vi "Controller List.vi"(11 "Controller List":T1[](array[typedef])=[{"Controller Name"=enum."Kuhnke", "CommSeg"=1, "PWM?"=TRUE, "Frequency"=100, "Low Command"=10.0, "High Command"=100.0, "Stop Command"=10.0, "Command Step"=0.1, "Solenoid Stop?"=FALSE, "Controller?"=TRUE, "Invert PWM"=TRUE, "Flange Mount Ctrl"=FALSE, "Diagnostic Mode"=enum."None"}, {"Controller Name"=enum."Helbako BLDC", "CommSeg"=1, "PWM?"=TRUE, "Frequency"=100, "Low Command"=10.0, "High Command"=100.0, "Stop Command"=10.0, "Command Step"=0.1, "Solenoid Stop?"=FALSE, "Controller?"=TRUE, "Invert PWM"=TRUE, "Flange Mount Ctrl"=FALSE, "Diagnostic Mode"=enum."None"}, {"Controller Name"=enum."Conti", "CommSeg"=1, "PWM?"=FALSE, "Frequency"=100, "Low Command"=0.0, "High Command"=800.0, "Stop Command"=0.0, "Command Step"=1.0, "Solenoid Stop?"=FALSE, "Controller?"=TRUE, "Invert PWM"=FALSE, "Flange Mount Ctrl"=FALSE, "Diagnostic Mode"=enum."None"}, {"Controller Name"=enum."Hella BLDC OL PWM", "CommSeg"=1, "PWM?"=FALSE, "Frequency"=100, "Low Command"=0.0, "High Command"=100.0, "Stop Command"=0.0, "Command Step"=0.1, "Solenoid Stop?"=FALSE, "Controller?"=TRUE, "Invert PWM"=FALSE, "Flange Mount Ctrl"=FALSE, "Diagnostic Mode"=enum."None"}, {"Controller Name"=enum."Hella BLDC Turbine OL PWM", "CommSeg"=1, "PWM?"=FALSE, "Frequency"=100, "Low Command"=0.0, "High Command"=100.0, "Stop Command"=0.0, "Command Step"=0.1, "Solenoid Stop?"=FALSE, "Controller?"=TRUE, "Invert PWM"=FALSE, "Flange Mount Ctrl"=FALSE, "Diagnostic Mode"=enum."None"}, {"Controller Name"=enum."Hella BLDC Pressure", "CommSeg"=1, "PWM?"=FALSE, "Frequency"=100, "Low Command"=0.0, "High Command"=100.0, "Stop Command"=0.0, "Command Step"=0.1, "Solenoid Stop?"=FALSE, "Controller?"=TRUE, "Invert PWM"=FALSE, "Flange Mount Ctrl"=FALSE, "Diagnostic Mode"=enum."None"}, {"Controller Name"=enum."Helbako (old)", "CommSeg"=1, "PWM?"=FALSE, "Frequency"=100, "Low Command"=0.0, "High Command"=100.0, "Stop Command"=0.0, "Command Step"=0.1, "Solenoid Stop?"=FALSE, "Controller?"=TRUE, "Invert PWM"=FALSE, "Flange Mount Ctrl"=FALSE, "Diagnostic Mode"=enum."None"}, {"Controller Name"=enum."TI PWM", "CommSeg"=1, "PWM?"=TRUE, "Frequency"=100, "Low Command"=0.0, "High Command"=100.0, "Stop Command"=0.0, "Command Step"=0.1, "Solenoid Stop?"=FALSE, "Controller?"=TRUE, "Invert PWM"=FALSE, "Flange Mount Ctrl"=FALSE, "Diagnostic Mode"=enum."None"}, {"Controller Name"=enum."PSA", "CommSeg"=1, "PWM?"=TRUE, "Frequency"=100, "Low Command"=5.0, "High Command"=95.0, "Stop Command"=5.0, "Command Step"=0.1, "Solenoid Stop?"=FALSE, "Controller?"=TRUE, "Invert PWM"=TRUE, "Flange Mount Ctrl"=TRUE, "Diagnostic Mode"=enum."PSA"}, {"Controller Name"=enum."Hella Gas", "CommSeg"=1, "PWM?"=FALSE, "Frequency"=100, "Low Command"=0.0, "High Command"=800.0, "Stop Command"=0.0, "Command Step"=1.0, "Solenoid Stop?"=TRUE, "Controller?"=TRUE, "Invert PWM"=FALSE, "Flange Mount Ctrl"=FALSE, "Diagnostic Mode"=enum."None"}, {"Controller Name"=enum."Hella Diesel", "CommSeg"=1, "PWM?"=FALSE, "Frequency"=100, "Low Command"=370.0, "High Command"=461.0, "Stop Command"=370.0, "Command Step"=1.0, "Solenoid Stop?"=TRUE, "Controller?"=TRUE, "Invert PWM"=FALSE, "Flange Mount Ctrl"=FALSE, "Diagnostic Mode"=enum."None"}, {"Controller Name"=enum."8 Comm", "CommSeg"=4, "PWM?"=FALSE, "Frequency"=100, "Low Command"=0.0, "High Command"=1.0, "Stop Command"=0.0, "Command Step"=1.0, "Solenoid Stop?"=FALSE, "Controller?"=FALSE, "Invert PWM"=FALSE, "Flange Mount Ctrl"=FALSE, "Diagnostic Mode"=enum."None"}, {"Controller Name"=enum."10 Comm", "CommSeg"=5, "PWM?"=FALSE, "Frequency"=100, "Low Command"=0.0, "High Command"=1.0, "Stop Command"=0.0, "Command Step"=1.0, "Solenoid Stop?"=FALSE, "Controller?"=FALSE, "Invert PWM"=FALSE, "Flange Mount Ctrl"=FALSE, "Diagnostic Mode"=enum."None"}, {"Controller Name"=enum."8 Comm Hella", "CommSeg"=4, "PWM?"=TRUE, "Frequency"=150, "Low Command"=0.0, "High Command"=50.0, "Stop Command"=80.0, "Command Step"=0.1, "Solenoid Stop?"=FALSE, "Controller?"=TRUE, "Invert PWM"=FALSE, "Flange Mount Ctrl"=FALSE, "Diagnostic Mode"=enum."None"}, {"Controller Name"=enum."10 Comm Hella", "CommSeg"=5, "PWM?"=TRUE, "Frequency"=150, "Low Command"=0.0, "High Command"=50.0, "Stop Command"=80.0, "Command Step"=0.1, "Solenoid Stop?"=FALSE, "Controller?"=TRUE, "Invert PWM"=FALSE, "Flange Mount Ctrl"=FALSE, "Diagnostic Mode"=enum."None"}, {"Controller Name"=enum."8 Comm Omron", "CommSeg"=4, "PWM?"=TRUE, "Frequency"=150, "Low Command"=5.0, "High Command"=50.0, "Stop Command"=75.0, "Command Step"=0.1, "Solenoid Stop?"=FALSE, "Controller?"=TRUE, "Invert PWM"=FALSE, "Flange Mount Ctrl"=FALSE, "Diagnostic Mode"=enum."None"}, {"Controller Name"=enum."10 Comm Omron", "CommSeg"=5, "PWM?"=TRUE, "Frequency"=150, "Low Command"=5.0, "High Command"=50.0, "Stop Command"=75.0, "Command Step"=0.1, "Solenoid Stop?"=FALSE, "Controller?"=TRUE, "Invert PWM"=FALSE, "Flange Mount Ctrl"=FALSE, "Diagnostic Mode"=enum."None"}, {"Controller Name"=enum."8 Comm Nissan", "CommSeg"=4, "PWM?"=TRUE, "Frequency"=10, "Low Command"=50.0, "High Command"=90.0, "Stop Command"=50.0, "Command Step"=0.1, "Solenoid Stop?"=TRUE, "Controller?"=TRUE, "Invert PWM"=FALSE, "Flange Mount Ctrl"=FALSE, "Diagnostic Mode"=enum."None"}, {"Controller Name"=enum."10 Comm Nissan", "CommSeg"=5, "PWM?"=TRUE, "Frequency"=10, "Low Command"=50.0, "High Command"=90.0, "Stop Command"=50.0, "Command Step"=0.1, "Solenoid Stop?"=TRUE, "Controller?"=TRUE, "Invert PWM"=FALSE, "Flange Mount Ctrl"=FALSE, "Diagnostic Mode"=enum."None"}, {"Controller Name"=enum."8 Comm Hella (for FCA)", "CommSeg"=4, "PWM?"=TRUE, "Frequency"=150, "Low Command"=11.0, "High Command"=89.0, "Stop Command"=10.0, "Command Step"=0.1, "Solenoid Stop?"=FALSE, "Controller?"=TRUE, "Invert PWM"=TRUE, "Flange Mount Ctrl"=FALSE, "Diagnostic Mode"=enum."None"}, {"Controller Name"=enum."Mazda BLDC", "CommSeg"=1, "PWM?"=TRUE, "Frequency"=250, "Low Command"=10.0, "High Command"=90.0, "Stop Command"=5.0, "Command Step"=0.1, "Solenoid Stop?"=FALSE, "Controller?"=TRUE, "Invert PWM"=TRUE, "Flange Mount Ctrl"=FALSE, "Diagnostic Mode"=enum."None"}, {"Controller Name"=enum."CMFB", "CommSeg"=1, "PWM?"=TRUE, "Frequency"=250, "Low Command"=0.0, "High Command"=100.0, "Stop Command"=10.0, "Command Step"=0.1, "Solenoid Stop?"=FALSE, "Controller?"=TRUE, "Invert PWM"=TRUE, "Flange Mount Ctrl"=TRUE, "Diagnostic Mode"=enum."CMFB"}]) -> (3 "Controller List OUT":T1[](array[typedef])=[{"Controller Name"=enum."Kuhnke", "CommSeg"=1, "PWM?"=TRUE, "Frequency"=100, "Low Command"=10.0, "High Command"=100.0, "Stop Command"=10.0, "Command Step"=0.1, "Solenoid Stop?"=FALSE, "Controller?"=TRUE, "Invert PWM"=TRUE, "Flange Mount Ctrl"=FALSE, "Diagnostic Mode"=enum."None"}, {"Controller Name"=enum."Helbako BLDC", "CommSeg"=1, "PWM?"=TRUE, "Frequency"=100, "Low Command"=10.0, "High Command"=100.0, "Stop Command"=10.0, "Command Step"=0.1, "Solenoid Stop?"=FALSE, "Controller?"=TRUE, "Invert PWM"=TRUE, "Flange Mount Ctrl"=FALSE, "Diagnostic Mode"=enum."None"}, {"Controller Name"=enum."Conti", "CommSeg"=1, "PWM?"=FALSE, "Frequency"=100, "Low Command"=0.0, "High Command"=800.0, "Stop Command"=0.0, "Command Step"=1.0, "Solenoid Stop?"=FALSE, "Controller?"=TRUE, "Invert PWM"=FALSE, "Flange Mount Ctrl"=FALSE, "Diagnostic Mode"=enum."None"}, {"Controller Name"=enum."Hella BLDC OL PWM", "CommSeg"=1, "PWM?"=FALSE, "Frequency"=100, "Low Command"=0.0, "High Command"=100.0, "Stop Command"=0.0, "Command Step"=0.1, "Solenoid Stop?"=FALSE, "Controller?"=TRUE, "Invert PWM"=FALSE, "Flange Mount Ctrl"=FALSE, "Diagnostic Mode"=enum."None"}, {"Controller Name"=enum."Hella BLDC Turbine OL PWM", "CommSeg"=1, "PWM?"=FALSE, "Frequency"=100, "Low Command"=0.0, "High Command"=100.0, "Stop Command"=0.0, "Command Step"=0.1, "Solenoid Stop?"=FALSE, "Controller?"=TRUE, "Invert PWM"=FALSE, "Flange Mount Ctrl"=FALSE, "Diagnostic Mode"=enum."None"}, {"Controller Name"=enum."Hella BLDC Pressure", "CommSeg"=1, "PWM?"=FALSE, "Frequency"=100, "Low Command"=0.0, "High Command"=100.0, "Stop Command"=0.0, "Command Step"=0.1, "Solenoid Stop?"=FALSE, "Controller?"=TRUE, "Invert PWM"=FALSE, "Flange Mount Ctrl"=FALSE, "Diagnostic Mode"=enum."None"}, {"Controller Name"=enum."Helbako (old)", "CommSeg"=1, "PWM?"=FALSE, "Frequency"=100, "Low Command"=0.0, "High Command"=100.0, "Stop Command"=0.0, "Command Step"=0.1, "Solenoid Stop?"=FALSE, "Controller?"=TRUE, "Invert PWM"=FALSE, "Flange Mount Ctrl"=FALSE, "Diagnostic Mode"=enum."None"}, {"Controller Name"=enum."TI PWM", "CommSeg"=1, "PWM?"=TRUE, "Frequency"=100, "Low Command"=0.0, "High Command"=100.0, "Stop Command"=0.0, "Command Step"=0.1, "Solenoid Stop?"=FALSE, "Controller?"=TRUE, "Invert PWM"=FALSE, "Flange Mount Ctrl"=FALSE, "Diagnostic Mode"=enum."None"}, {"Controller Name"=enum."PSA", "CommSeg"=1, "PWM?"=TRUE, "Frequency"=100, "Low Command"=5.0, "High Command"=95.0, "Stop Command"=5.0, "Command Step"=0.1, "Solenoid Stop?"=FALSE, "Controller?"=TRUE, "Invert PWM"=FALSE, "Flange Mount Ctrl"=FALSE, "Diagnostic Mode"=enum."None"}, {"Controller Name"=enum."Hella Gas", "CommSeg"=1, "PWM?"=FALSE, "Frequency"=100, "Low Command"=0.0, "High Command"=800.0, "Stop Command"=0.0, "Command Step"=1.0, "Solenoid Stop?"=TRUE, "Controller?"=TRUE, "Invert PWM"=FALSE, "Flange Mount Ctrl"=FALSE, "Diagnostic Mode"=enum."None"}, {"Controller Name"=enum."Hella Diesel", "CommSeg"=1, "PWM?"=FALSE, "Frequency"=100, "Low Command"=370.0, "High Command"=461.0, "Stop Command"=370.0, "Command Step"=1.0, "Solenoid Stop?"=TRUE, "Controller?"=TRUE, "Invert PWM"=FALSE, "Flange Mount Ctrl"=FALSE, "Diagnostic Mode"=enum."None"}, {"Controller Name"=enum."8 Comm", "CommSeg"=4, "PWM?"=FALSE, "Frequency"=100, "Low Command"=0.0, "High Command"=1.0, "Stop Command"=0.0, "Command Step"=1.0, "Solenoid Stop?"=FALSE, "Controller?"=FALSE, "Invert PWM"=FALSE, "Flange Mount Ctrl"=FALSE, "Diagnostic Mode"=enum."None"}, {"Controller Name"=enum."10 Comm", "CommSeg"=5, "PWM?"=FALSE, "Frequency"=100, "Low Command"=0.0, "High Command"=1.0, "Stop Command"=0.0, "Command Step"=1.0, "Solenoid Stop?"=FALSE, "Controller?"=FALSE, "Invert PWM"=FALSE, "Flange Mount Ctrl"=FALSE, "Diagnostic Mode"=enum."None"}, {"Controller Name"=enum."8 Comm Hella", "CommSeg"=4, "PWM?"=TRUE, "Frequency"=150, "Low Command"=0.0, "High Command"=50.0, "Stop Command"=80.0, "Command Step"=0.1, "Solenoid Stop?"=FALSE, "Controller?"=TRUE, "Invert PWM"=FALSE, "Flange Mount Ctrl"=FALSE, "Diagnostic Mode"=enum."None"}, {"Controller Name"=enum."10 Comm Hella", "CommSeg"=5, "PWM?"=TRUE, "Frequency"=150, "Low Command"=0.0, "High Command"=50.0, "Stop Command"=80.0, "Command Step"=0.1, "Solenoid Stop?"=FALSE, "Controller?"=TRUE, "Invert PWM"=FALSE, "Flange Mount Ctrl"=FALSE, "Diagnostic Mode"=enum."None"}, {"Controller Name"=enum."8 Comm Omron", "CommSeg"=4, "PWM?"=TRUE, "Frequency"=150, "Low Command"=5.0, "High Command"=50.0, "Stop Command"=75.0, "Command Step"=0.1, "Solenoid Stop?"=FALSE, "Controller?"=TRUE, "Invert PWM"=FALSE, "Flange Mount Ctrl"=FALSE, "Diagnostic Mode"=enum."None"}, {"Controller Name"=enum."10 Comm Omron", "CommSeg"=5, "PWM?"=TRUE, "Frequency"=150, "Low Command"=5.0, "High Command"=50.0, "Stop Command"=75.0, "Command Step"=0.1, "Solenoid Stop?"=FALSE, "Controller?"=TRUE, "Invert PWM"=FALSE, "Flange Mount Ctrl"=FALSE, "Diagnostic Mode"=enum."None"}, {"Controller Name"=enum."8 Comm Nissan", "CommSeg"=4, "PWM?"=TRUE, "Frequency"=10, "Low Command"=50.0, "High Command"=90.0, "Stop Command"=50.0, "Command Step"=0.1, "Solenoid Stop?"=TRUE, "Controller?"=TRUE, "Invert PWM"=FALSE, "Flange Mount Ctrl"=FALSE, "Diagnostic Mode"=enum."None"}, {"Controller Name"=enum."10 Comm Nissan", "CommSeg"=5, "PWM?"=TRUE, "Frequency"=10, "Low Command"=50.0, "High Command"=90.0, "Stop Command"=50.0, "Command Step"=0.1, "Solenoid Stop?"=TRUE, "Controller?"=TRUE, "Invert PWM"=FALSE, "Flange Mount Ctrl"=FALSE, "Diagnostic Mode"=enum."None"}])   [LabVIEW 2019]
uses:
  Controls/Controller Config.ctl
  Type Defs/Controller Names.ctl
  Type Defs/Diagnostic Mode.ctl
panel:
  # "Do a \"Make Values Default\" after making changes!!!!!"
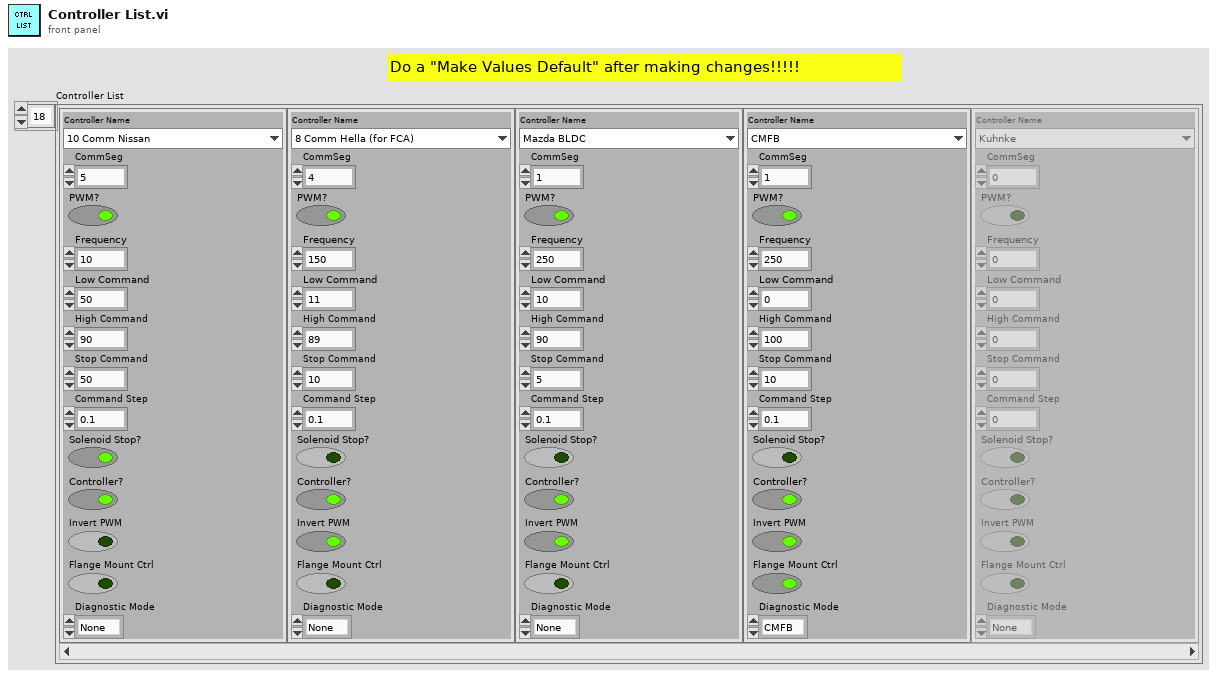
[diagram p1: front panel]
types:
  T1 = typedef "Controller Config.ctl" = cluster{"Controller Name":T2, "CommSeg":i32, "PWM?":bool, "Frequency":i32, "Low Command":dbl, "High Command":dbl, "Stop Command":dbl, "Command Step":dbl, "Solenoid Stop?":bool, "Controller?":bool, "Invert PWM":bool, "Flange Mount Ctrl":bool, "Diagnostic Mode":T3}
  T2 = typedef "Controller Names.ctl" = enum16{"Kuhnke", "Helbako BLDC", "Conti", "Hella BLDC OL PWM", "Hella BLDC Turbine OL PWM", "Hella BLDC Pressure", "Helbako (old)", "TI PWM", "PSA", "Hella Gas", "Hella Diesel", "8 Comm", "10 Comm", "8 Comm Hella", "10 Comm Hella", "8 Comm Omron", "10 Comm Omron", "8 Comm Nissan", "10 Comm Nissan", "8 Comm Hella (for FCA)", "Mazda BLDC", "CMFB"}
  T3 = typedef "Diagnostic Mode.ctl" = enum16{"None", "PSA", "CMFB"}
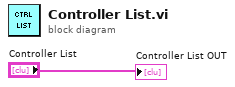
[diagram p0: block diagram]
diagram:
  "Controller List OUT" <- "Controller List"
